vi "Init LCD.vi"(8 "error in (no error)":errorcluster, 11 "PCF8574 I2C LCD in":refnum<class "PCF8574 I2C LCD.lvclass">) -> (0 "error out":errorcluster, 3 "PCF8574 I2C LCD out":refnum<class "PCF8574 I2C LCD.lvclass">)   [LabVIEW 2020, in "CTI-Peripheral.lvlib" / "PCF8574 I2C LCD.lvclass"]
uses:
  PCF8574 I2C LCD.lvclass
  PCF8574 I2C LCD.lvclass/PCF8574 I2C LCD.ctl
  Character LCD/Entry Shift.ctl
  Character LCD/Char LCD.lvclass
  Character LCD/Glyph Entry.ctl
  HD44780 LCD/Display Mode.ctl
  HD44780 LCD/HD44780 LCD.lvlib
  Character LCD/Bus Mode.ctl
  Character LCD/Lines.ctl
  Character LCD/Glyph Size.ctl
  HD44780 LCD/Display Function.ctl
  HD44780 LCD/Display Control.ctl
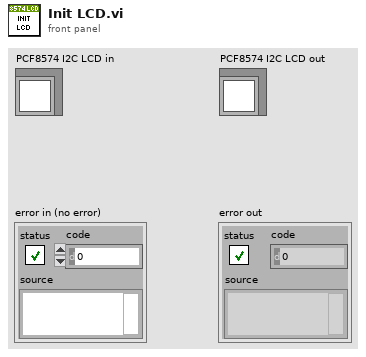
[diagram p1: front panel]
types:
  T1 = typedef "CTI-Peripheral.lvlib/HD44780 LCD.lvlib/Display Control.ctl" = cluster{"Blink On":bool, "Cursor On":bool, "Display On":bool}
  T2 = typedef "CTI-Peripheral.lvlib/HD44780 LCD.lvlib/Display Function.ctl" = cluster{"Bus Mode":T3, "Lines":T4, "Glyph Size":T5}
  T3 = typedef "CTI-Peripheral.lvlib/Char LCD.lvclass/Bus Mode.ctl" = enum8{"4 Bit", "8 Bit"}
  T4 = typedef "CTI-Peripheral.lvlib/Char LCD.lvclass/Lines.ctl" = enum8{"Single", "Multiline"}
  T5 = typedef "CTI-Peripheral.lvlib/Char LCD.lvclass/Glyph Size.ctl" = enum8{"5x8", "5x10"}
  T6 = typedef "CTI-Peripheral.lvlib/HD44780 LCD.lvlib/Display Mode.ctl" = cluster{"Entry Shift":T7, "Glyph Entry":T8}
  T7 = typedef "CTI-Peripheral.lvlib/Char LCD.lvclass/Entry Shift.ctl" = enum8{"Decrement", "Increment"}
  T8 = typedef "CTI-Peripheral.lvlib/Char LCD.lvclass/Glyph Entry.ctl" = enum8{"Right", "Left"}
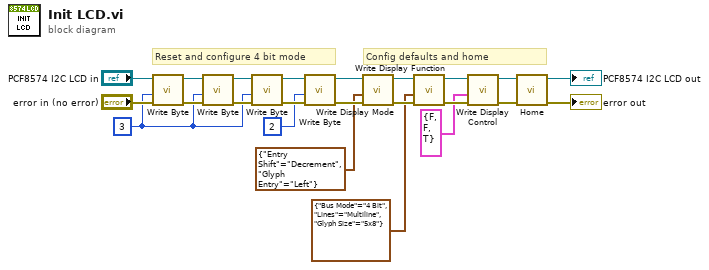
[diagram p0: block diagram]
diagram:
  w17 = u8 3 ("Value")
  # "Config defaults and home"
  # "Reset and configure 4 bit mode"
  n1 = call "Write Byte.vi"("error in (no error)"="error in (no error)", "Value"=w17, "PCF8574 I2C LCD in"="PCF8574 I2C LCD in") -> ("error out"=w20:errorcluster, "PCF8574 I2C LCD out"=w21:refnum<class "PCF8574 I2C LCD.lvclass">)  [unwired: 7 in]
  n2 = call "Write Byte.vi"("error in (no error)"=w20, "Value"=w17, "PCF8574 I2C LCD in"=w21) -> ("error out"=w19:errorcluster, "PCF8574 I2C LCD out"=w18:refnum<class "PCF8574 I2C LCD.lvclass">)  [unwired: 7 in]
  n3 = call "Write Byte.vi"("error in (no error)"=w19, "Value"=w17, "PCF8574 I2C LCD in"=w18) -> ("error out"=w16:errorcluster, "PCF8574 I2C LCD out"=w15:refnum<class "PCF8574 I2C LCD.lvclass">)  [unwired: 7 in]
  n4 = call "Write Byte.vi"("error in (no error)"=w16, "Value"=u8 2, "PCF8574 I2C LCD in"=w15) -> ("error out"=w12:errorcluster, "PCF8574 I2C LCD out"=w13:refnum<class "PCF8574 I2C LCD.lvclass">)  [unwired: 7 in]
  n5 = call "Write Display Mode.vi"("error in (no error)"=w12, "Display Mode"=T6 {"Entry Shift"=enum."Decrement", "Glyph Entry"=enum."Left"}, "PCF8574 I2C LCD in"=w13) -> ("error out"=w9:errorcluster, "PCF8574 I2C LCD out"=w10:refnum<class "PCF8574 I2C LCD.lvclass">)  [unwired: 7 in]
  n6 = call "Write Display Function.vi"("error in (no error)"=w9, "Display Function"=T2 {"Bus Mode"=enum."4 Bit", "Lines"=enum."Multiline", "Glyph Size"=enum."5x8"}, "PCF8574 I2C LCD in"=w10) -> ("error out"=w7:errorcluster, "PCF8574 I2C LCD out"=w6:refnum<class "PCF8574 I2C LCD.lvclass">)  [unwired: 7 in]
  n7 = call "Write Display Control.vi"("error in (no error)"=w7, "Display Control"=T1 {"Blink On"=FALSE, "Cursor On"=FALSE, "Display On"=TRUE}, "PCF8574 I2C LCD in"=w6) -> ("error out"=w4:errorcluster, "PCF8574 I2C LCD out"=w3:refnum<class "PCF8574 I2C LCD.lvclass">)  [unwired: 7 in]
  n8 = call-dynamic "Home.vi"("error in (no error)"=w4, "Character LCD in"=w3) -> ("error out"=→"error out":errorcluster, "Character LCD out"=→"PCF8574 I2C LCD out":refnum<class "PCF8574 I2C LCD.lvclass">)  [unwired: 8 in]
